vi "cs-scanning_v4_ssx.vi"() -> ()   [LabVIEW 2017]
uses:
  controls/boolean_info.ctl
  controls/z-axis-params_v4_prescan.ctl
  controls/TF-params.ctl
  fpga_subVIs_ssxy/fixed-point-ss/typeDefs/FXPControlParams_distEst.ctl
  <vilib>/Platform/TimedLoop/XDataNode/timing_clust.ctl
  <vilib>/Platform/TimedLoop/XDataNode/nitl_modes.ctl
  <vilib>/Platform/TimedLoop/XDataNode/wakeup.ctl
  <vilib>/rvi/Emulation/niFpgaSctlEmulationGetInTimedLoop.vi
  <vilib>/rvi/Emulation/niFpgaProcessEmulError.vi
  <vilib>/rvi/Emulation/niFpgaEmulationReportErrorSimple.vi
  <vilib>/rvi/Emulation/niFpgaGetClockAttributes.vi
  <vilib>/rvi/Emulation/niFpgaCriticalErrorInLSC.vi
  <vilib>/rvi/Memory/Memory_Emulation/nirvimemoryFastEmulation.vi
  <vilib>/rvi/Memory/Memory_Emulation/nirvimemoryEmulation.vi
  <vilib>/rvi/Emulation/niFpgaEmulationIsFPGAContextNoSignature.vi
  <vilib>/rvi/DataTransferAndStorage/Container/Common/niFpgaContainerGetUniqueNameForEmu.vi
  <vilib>/rvi/errors/nirviReportUnexpectedCaseInternalError (U32).vi
  <vilib>/rvi/eio/common/nirviEmuTemplateMethod_errors.vi
  <vilib>/rvi/Memory/Memory_Emulation/niFpgaMemoryEmulationCacheClearOnFirstRun.vi
  <vilib>/rvi/Memory/Memory_Emulation/nirvimemoryEmulationManagerCache_MakeExclusive.vi
  <vilib>/rvi/Memory/Memory_Emulation/niFpgaMemoryEmulationValidateCache.vi
  <vilib>/rvi/Memory/Memory_Emulation/nirvimemoryEmulationManagerCache_InsertValue.vi
  <vilib>/Utility/error.llb/Clear Errors.vi
  <vilib>/rvi/Memory/Memory_Emulation/nirvimemoryEmulationManagerCache_ReleaseExclusive.vi
  <vilib>/rvi/Memory/Memory_Emulation/nirvimemoryEmulationManagerCache_GetValue.vi
  <vilib>/rvi/Memory/Memory_Emulation/nirvimemoryEmulationManagerCache_SetValue.vi
  <vilib>/Platform/TimedLoop/XDataNode/XDataNode.xnode
  <vilib>/rvi/DataTransferAndStorage/Container/XNode/niFpgaContainer.xnode
  <vilib>/eio/EIONode/EIONode.xnode
  <vilib>/rvi/DataTransferAndStorage/Register/Emulation/niFpgaRegisterEmulation.vi
  FPGA-data-logging.lvlib
  libimaging-cs.lvlib
  <vilib>/Platform/TimedLoop/XDataNode/XDNodeRunTimeDep.lvlib
panel:
  in  "num-log-channels":i32
  out "SS FIFO TimeOut?":bool
  in  "ControlParamsLin":T1={"umax"=3.0, "Ns_obs/cntrl"=0, "ref_f_VEC"=[0.0, 0.0], "du_max"=0.0, "Nbar"=0.0, "Nhyst"=0, "Nsat"=0, "Ndrift+1"=0}
  in  "z_axis_params":T2={"TOL"=0.3, "z_u_max"=5.0, "setpoint-scan"=0.0, "Ki-scan"=0.001, "uz_safe"=0.0, "Kiz_down"=0.001, "prescan-samples"=0, "setpoint-up"=0.0, "TF-params"={"TF-order"=0, "Num"=[0.0, 0.0, 0.0, 0.0, 0.0, 0.0, 0.0, 0.0, 0.0], "Den"=[0.0, 0.0, 0.0, 0.0, 0.0, 0.0, 0.0, 0.0, 0.0]}, "do-Dz"=FALSE, "PID-while-xy-move"=FALSE} {"prescan-samples" format="%#_13g"; "uz_safe" format="%#_13g"; "TOL" format="%#_13g"}
  in  "zup-err-threshold":fxp<+,24,5>=0.10000038146972656 format="%#_21g"
  out "stop_loops":bool
  out "xy_k":fxp<+/-,16,5>[](array[numeric])
  out "xy_ref":fxp<+/-,16,5>[](array[numeric])
  out "u_x saturated":bool
  out "u_y saturated":bool
  out "state1-count":u64
  out "state5-count":u64
  out "state4-count":u64
  out "state3-count":u64
  out "state2-count":u64
  in  "collect all":bool
  out "entity-index":i16
  in  "TsTicks":u32=1600
  out "number-settled-samples-Z":i16
  out "Current Case":u8
  out "boolean \nindicators":T4
  out "z-u(k)":sgl
  in  "ABORT":bool
  out "read fifo timeout":bool
  in  "numEntities":i16
  in  "trigger-0":bool
  out "number-settled-samples-y":i16
  out "number-settled-samples-x":i16
  in  "xy-error-threshold":sgl format="%#_13g"
  in  "settled-samples\nthreshold":i16
  in  "Ki-xy":sgl=0.001 format="%#_13g"
  # "- If collect all = fasle ,\nwe only collect measurement data.\n- If collect all = true, we collect everything."
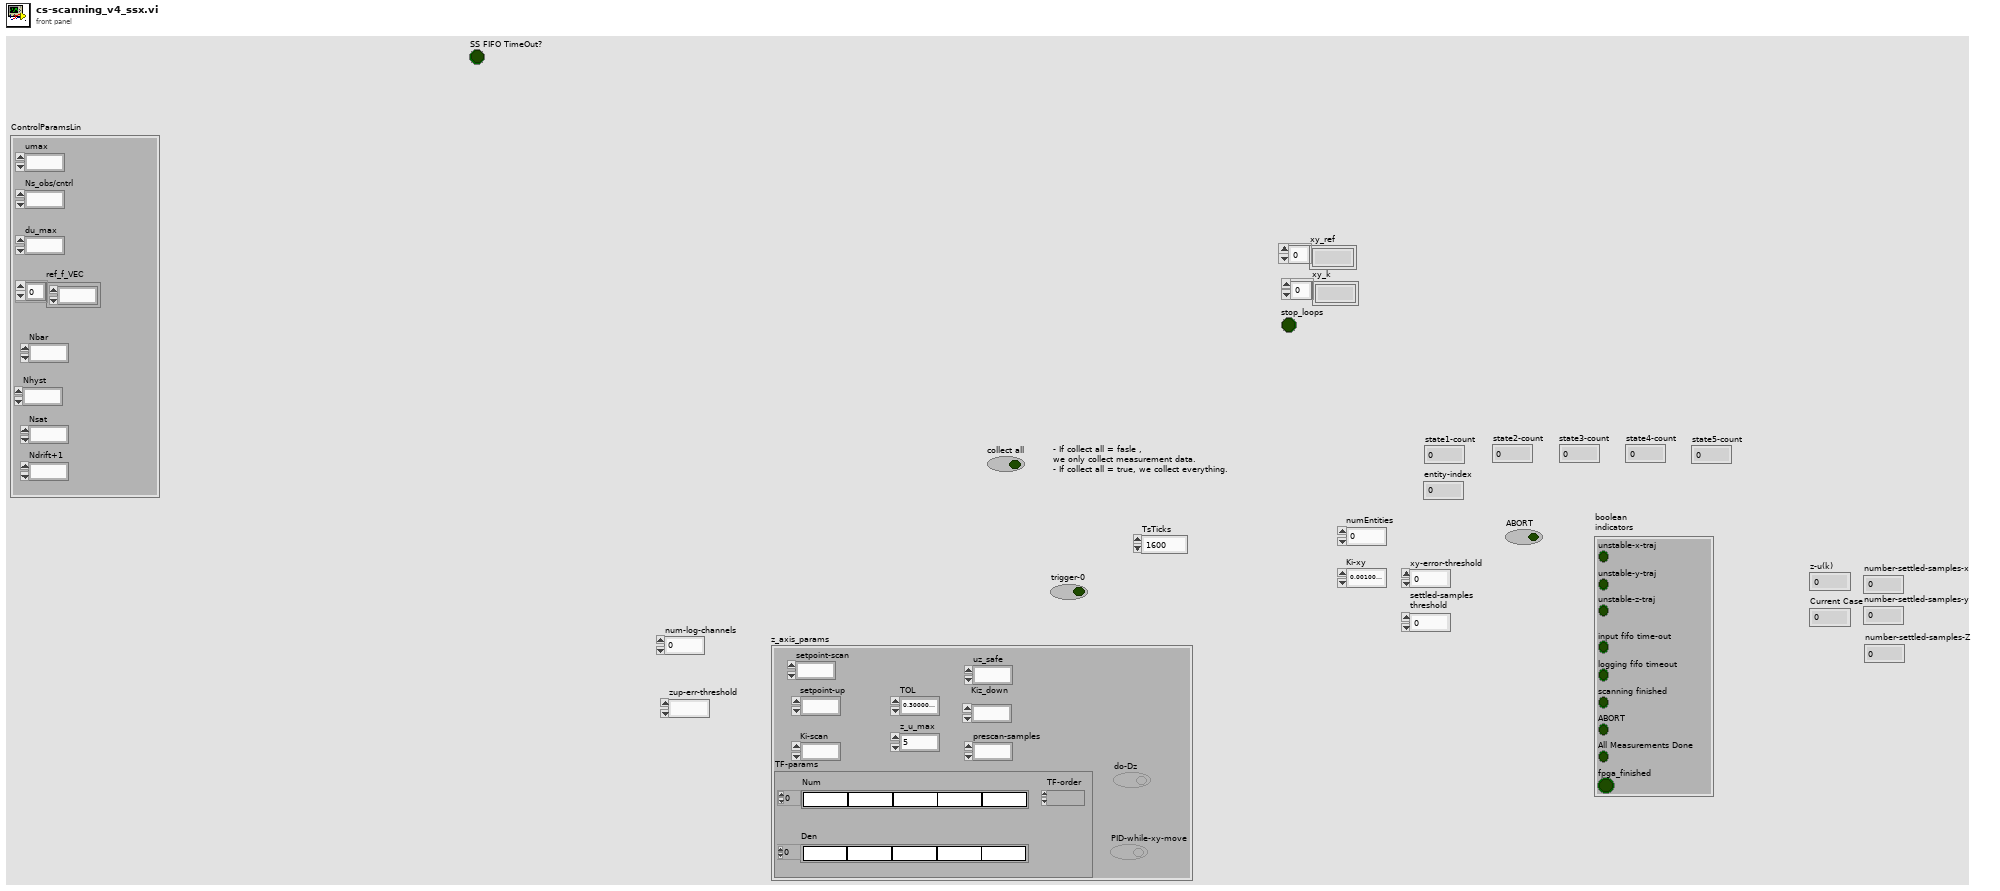
[diagram p1: front panel]
types:
  T1 = typedef "FXPControlParams_distEst.ctl" = cluster{"umax":fxp<+/-,18,5>, "Ns_obs/cntrl":u8, "ref_f_VEC":fxp<+/-,32,5>[], "du_max":fxp<+/-,18,5>, "Nbar":fxp<+/-,32,5>, "Nhyst":u8, "Nsat":u8, "Ndrift+1":u8}
  T2 = typedef "z-axis-params_v4_prescan.ctl" = cluster{"TOL":sgl, "z_u_max":sgl, "setpoint-scan":fxp<+/-,32,16>, "Ki-scan":sgl, "uz_safe":fxp<+/-,16,5>, "Kiz_down":sgl, "prescan-samples":i16, "setpoint-up":fxp<+/-,32,16>, "TF-params":T3, "do-Dz":bool, "PID-while-xy-move":bool}
  T3 = typedef "TF-params.ctl" = cluster{"TF-order":i16, "Num":sgl[], "Den":sgl[]}
  T4 = typedef "boolean_info.ctl" = cluster{"unstable-z-traj":bool, "input fifo time-out":bool, "logging fifo timeout":bool, "scanning finished":bool, "unstable-x-traj":bool, "unstable-y-traj":bool, "ABORT":bool, "All Measurements Done":bool, "fpga_finished":bool}
  T5 = typedef "XDNodeRunTimeDep.lvlib/timing_clust.ctl" = cluster{"Expected End [f-1]":u64, "Actual End [f-1]":u64, "Finished Late? [f-1]":bool, "Expected End [i-1]":u64, "Actual End [i-1]":u64, "Finished Late? [i-1]":bool, "Expected Start [i]":u64, "Actual Start [i]":u64, "Expected Start [f]":u64, "Actual Start [f]":u64, "Source Name":string, "Structure Name":string, "Period":i64, "Deadline":i64, "Offset":i64, "Start":i64, "Priority":i32, "Timeout":i32, "Mode":T6, "Wakeup Reason":T7, "Error":errorcluster, "Source Type":string, "Secondary Source Type":string, "Global End Time":u64, "Global Start Time":u64, "Frame Duration":u64, "Iteration Duration":u64, "Assigned CPU":i32, "I/O Scan Engine Mode":u32}
  T6 = typedef "XDNodeRunTimeDep.lvlib/nitl_modes.ctl" = enum32{"No Change", "Process missed periods, maintain original phase", "Discard missed periods, maintain original phase", "Process missed periods, ignore original phase", "Discard missed periods, ignore original phase"}
  T7 = typedef "XDNodeRunTimeDep.lvlib/wakeup.ctl" = enum32{"Normal", "Aborted", "Asynchronous wakeup", "Timing source error", "Timed loop error", "Timeout"}
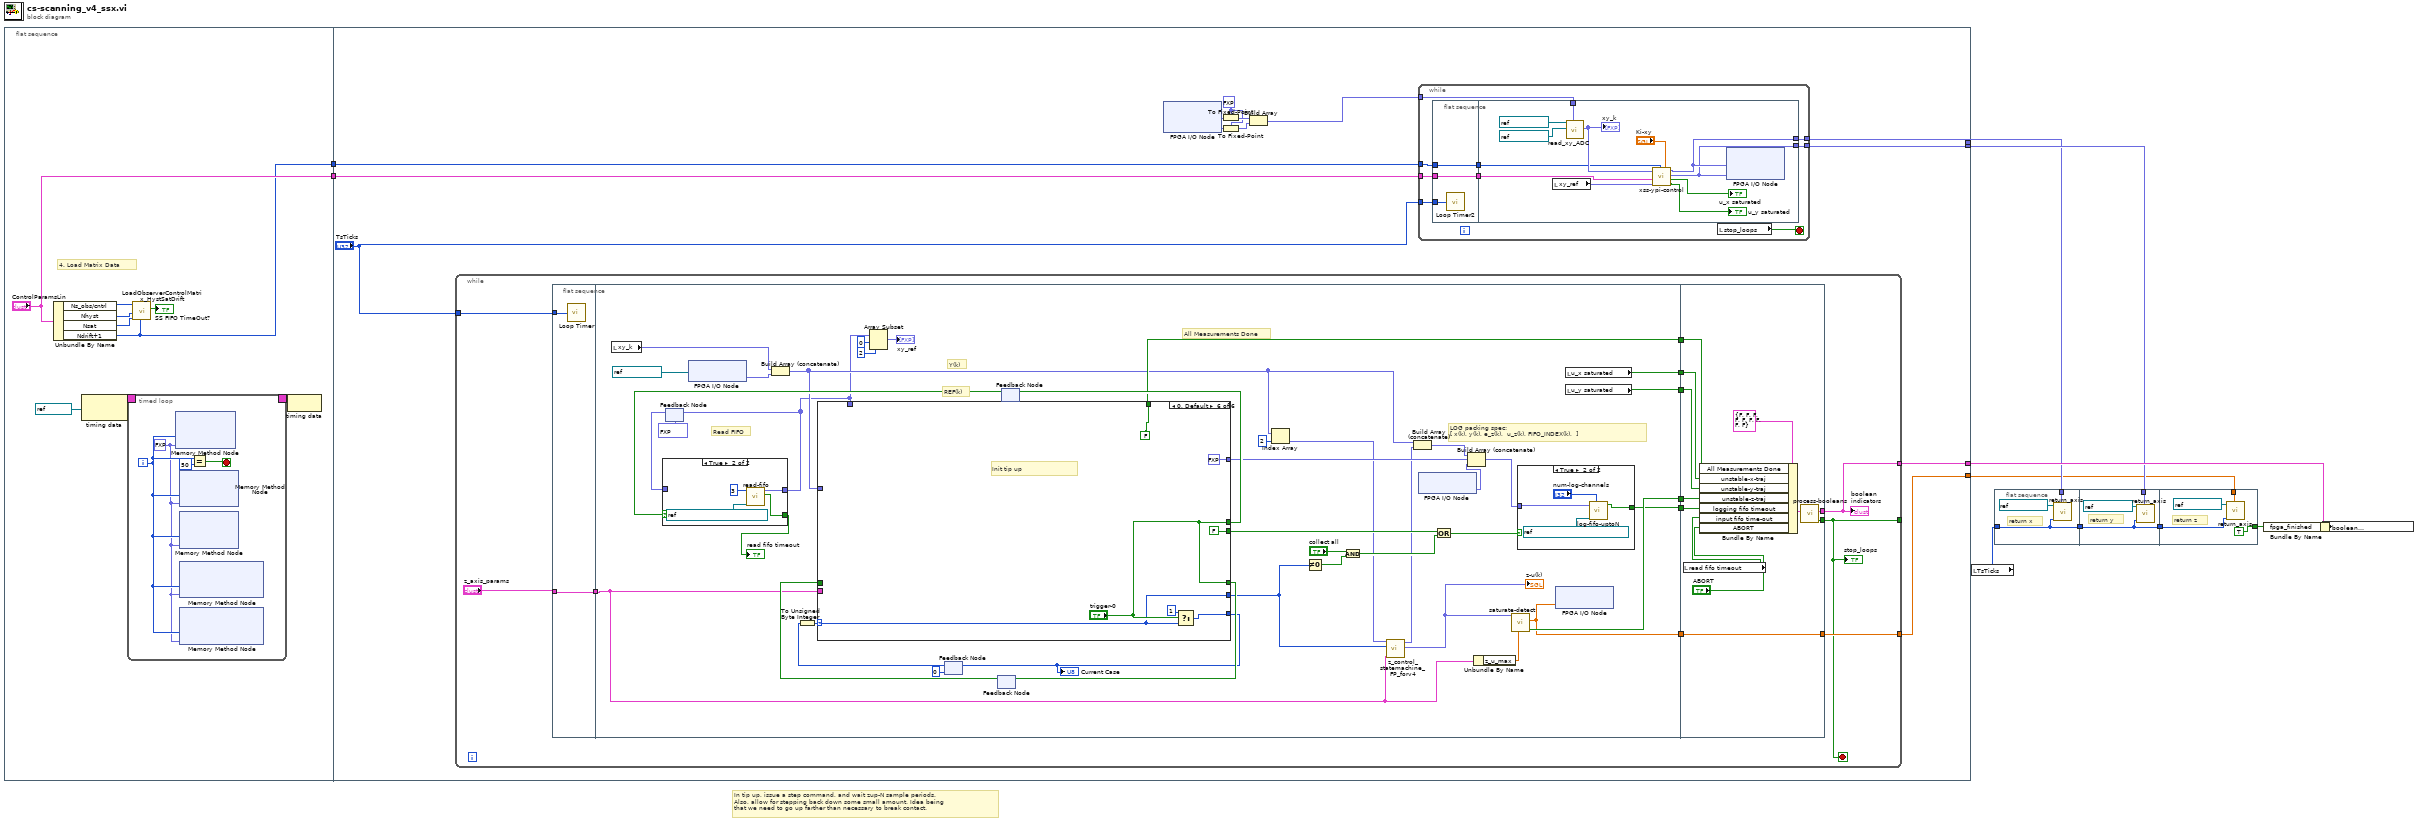
[diagram p0: block diagram]
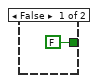
[diagram p2: hidden frame]
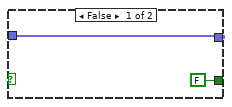
[diagram p3: hidden frame]
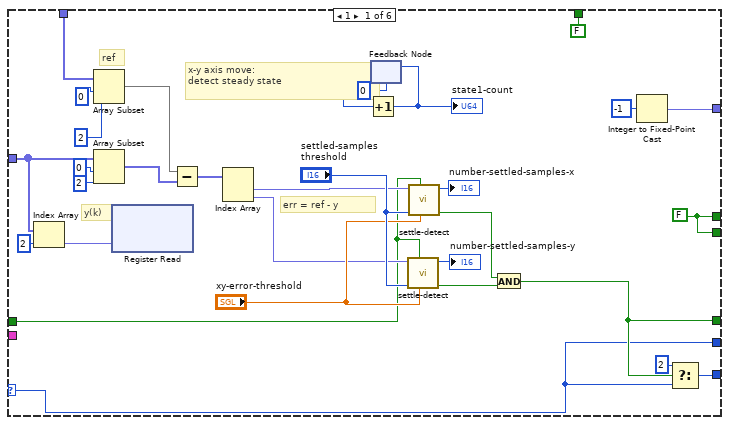
[diagram p4: hidden frame]
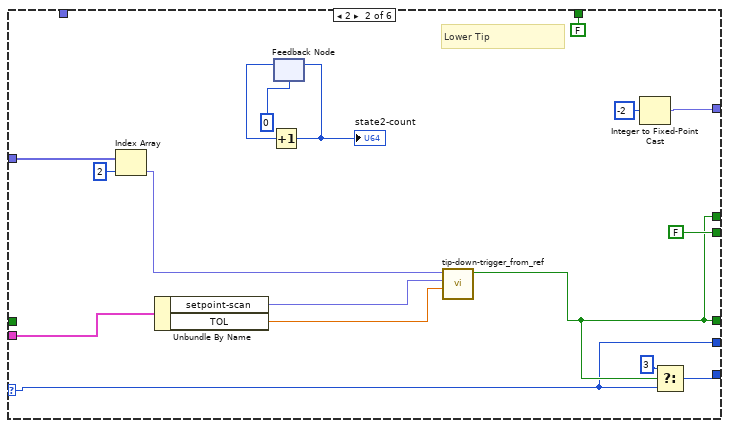
[diagram p5: hidden frame]
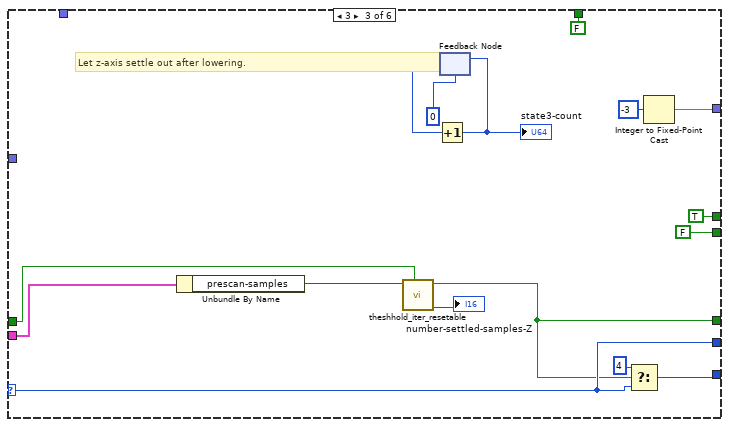
[diagram p6: hidden frame]
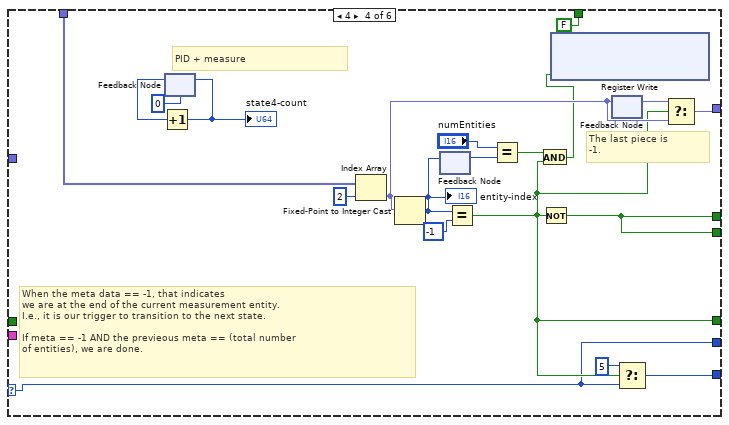
[diagram p7: hidden frame]
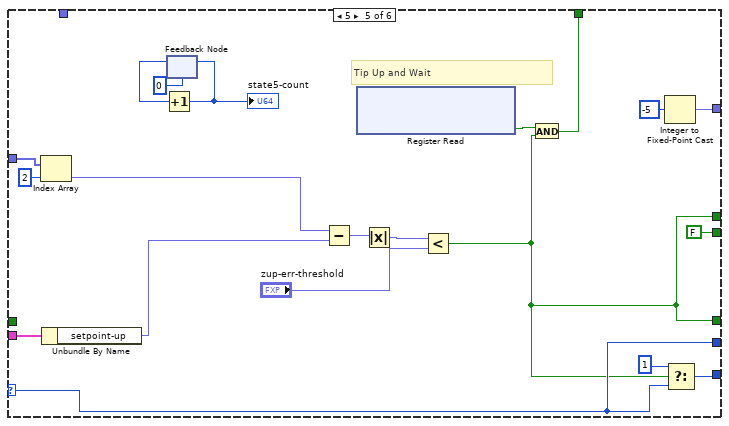
[diagram p8: hidden frame]
diagram:
  # "In tip up, issue a step command, and wait zup-N sample periods.\nAlso, allow for stepping back down some small amount. Idea being \nthat we need to go up farther than necessary to break contact."
  n1 = flat-sequence {
    tunnel: ["ControlParamsLin"] -> w2
    tunnel: [w12] -> w1
    tunnel: [w43] -> w9
    tunnel: [w41] -> w6
    tunnel: [w40] -> w5
    tunnel: [w39] -> w4
    tunnel: w2 -> [w32]
    tunnel: w1 -> [w31]
    frame #0 {
      # "4. Load Matrix Data"
      n2 = Unbundle By Name("ControlParamsLin") -> ("Ns_obs/cntrl"=w17:u8, "Nhyst"=w14:u8, "Nsat"=w13:u8, "Ndrift+1"=w12:u8)
      n3 = node-c288(refnum<k21> "80MHz" ("Source Name")) -> (w20:T5)
      n4 = timed-loop {
        timing: w20 -> [_]
        timing-out: [_] -> w19
        i -> [w22]
        stop <- w24 stop-if-true
        w21 = fxp<+/-,32,5> 0.0 ("Data")
        n5 = xnode ("Memory Method Node")("Address"=w22, "Data"=w21) -> ()  [unwired: 1 in, 1 out]
        n6 = xnode ("Memory Method Node")("Address"=w22, "Data"=w21) -> ()  [unwired: 1 in, 1 out]
        n7 = xnode ("Memory Method Node")("Address"=w22, "Data"=w21) -> ()  [unwired: 1 in, 1 out]
        n8 = xnode ("Memory Method Node")("Address"=w22, "Data"=w21) -> ()  [unwired: 1 in, 1 out]
        n9 = xnode ("Memory Method Node")("Address"=w22, "Data"=w21) -> ()  [unwired: 1 in, 1 out]
        n10 = Equal?(x=w22, y=50) -> (x = y?=w24:bool)
      }
      n11 = call "LoadObserverControlMatrix_HystSatDrift.vi"("Ndrift+1"=w12, "Nsat"=w13, "Nhyst"=w14, "NS_obs/cntrl"=w17) -> ("SS FIFO TimeOut?"=→"SS FIFO TimeOut?":bool)  [unwired: 7 in]
      n12 = node-c288(w19) -> ()
    }
    frame #1 {
      w34 = fxp<+/-,16,5> 0.0 ("fixed-point type")
      n13 = while {
        tunnel: "TsTicks" -> [w51]
        tunnel: [w47] -> _
        tunnel: [w49] -> w39
        tunnel: [w48] -> w43
        stop <- w47 stop-if-true
        n14 = flat-sequence {
          tunnel: w51 -> [w56]
          tunnel: "z_axis_params" -> [w57]
          tunnel: [w57] -> w55
          tunnel: w55 -> [w59]
          tunnel: [w96] -> w54
          tunnel: [w95] -> w53
          tunnel: [w83] -> w52
          tunnel: [w64] -> w50
          tunnel: [w78] -> w46
          tunnel: [w77] -> w45
          tunnel: w54 -> [w232]
          tunnel: w53 -> [w229]
          tunnel: w52 -> [w226]
          tunnel: [w225] -> w47
          tunnel: [w224] -> w48
          tunnel: [w223] -> w49
          tunnel: w50 -> [w223]
          tunnel: w46 -> [w222]
          tunnel: w45 -> [w221]
          frame #0 {
            n15 = call "Loop Timer"("Count(Ticks)"=w56) -> ()  [unwired: 1 out]
          }
          frame #1 {
            # "All Measurements Done"
            # "REF(k)"
            # "Y(k)"
            # "LOG packing spec:\n[ x(k), y(k), e_z(k),  u_z(k), FIFO_INDEX(k),  ]"
            # "Read FIFO"
            n16 = local read "xy_k"() -> (w70:fxp<+/-,16,5>[])
            n17 = feedback #1(fxp<+/-,16,5>[] [0.0, 0.0, 0.0] ("unpacked-data")) -> (w98:fxp<+/-,16,5>[])
            n18 = xnode "FPGA I/O Node"("FPGA I/O In"=refnum<k21> "Mod2/AI2" ("y - ADC")) -> ("I/O Item"=w74:fxp<+/-,24,5>)  [unwired: 1 out]
            n19 = Build Array (concatenate)(w70, w74) -> (w73:fxp<+/-,24,5>[])
            n20 = feedback #2(u8 0 ("t")) -> (w68:u8)
            n21 = To Unsigned Byte Integer(number=w68) -> (unsigned 8bit integer=w69:u8)
            n22 = feedback #3() -> (w89:bool)  [unwired: 1 in]
            n23 = feedback #4() -> (w92:bool)  [unwired: 1 in]
            n24 = case shown="True" w92 {
              tunnel: w98 -> [w105 _]
              tunnel: [w105 w107] -> w65
              tunnel: [FALSE ("timout?") w106] -> w94
              frame False {
              }
              frame True {
                n25 = call "read-fifo.vi"("FIFO In"=refnum<k21> "host-to-fpga-fxp-16-5", "numChan"=3) -> ("timout?"=w106:bool, "unpacked-data"=w107:fxp<+/-,16,5>[])  [unwired: 8 in]
              }
            }
            "read fifo timeout" <- w94
            n26 = feedback-in #1(w65) -> ()
            n27 = case shown="0, Default" w69 {
              selector: w69 -> [w110 w141 w162 w174 w201 w214]
              tunnel: [w111 FALSE FALSE ("trigger-0") w184 FALSE FALSE] -> w84
              tunnel: [w133 w153 w172 w192 w212 w220] -> w67
              tunnel: w73 -> [w112 w155 _ _ w203 _]
              tunnel: [w111 w143 TRUE ("trigger-0") w184 w196 "trigger-0"] -> w93
              tunnel: w59 -> [_ w157 w170 _ w195 _]
              tunnel: [FALSE FALSE FALSE FALSE w205 FALSE] -> w83
              tunnel: w65 -> [w124 _ _ w186 _ _]
              tunnel: w89 -> [w122 _ w163 _ _ _]
              tunnel: [w121 w143 w159 w177 w196 "trigger-0"] -> w90
              tunnel: [w115 w144 w164 w180 w206 fxp<+/-,16,5> 0.0 ("Element")] -> w71
              tunnel: [w110 w141 w162 w174 w201 w214] -> w62
              frame 1 {
                w111 = FALSE
                # "y(k)"
                # "err = ref - y"
                # "ref"
                # "x-y axis move: \ndetect steady state"
                n28 = Index Array(array=w112, index=2) -> (element=w114:fxp<+/-,24,5>)
                n29 = Array Subset(array=w124, index=0, length=2) -> (w128:fxp<+/-,16,5>[])
                n30 = Array Subset(array=w112, index=0, length=2) -> (w127:fxp<+/-,24,5>[])
                n31 = xnode ("Register Read")("Data"=w114) -> ()  [unwired: 1 in, 1 out]
                n32 = Subtract(x=w128, y=w127) -> (x-y=w120:fxp<+/-,25,6>[])
                n33 = Index Array(array=w120) -> (element #1=w126:fxp<+/-,25,6>, element #2=w125:fxp<+/-,25,6>)  [unwired: 2 in]
                n34 = feedback #5(u64 0) -> (w118:u64)
                n35 = Increment(x=w118) -> (x+1=w119:u64)
                "state1-count" <- w119
                n36 = feedback-in #5(w119) -> ()
                n37 = call "settle-detect.vi"("error-max"="xy-error-threshold", "reset"=w122, "settled-samples\nthreshold"="settled-samples\nthreshold", "err(k)"=w125) -> ("has-settled"=w140:bool, "number-settled-samples"=→"number-settled-samples-y":u16)  [unwired: 6 in]
                n38 = call "settle-detect.vi"("error-max"="xy-error-threshold", "reset"=w122, "settled-samples\nthreshold"="settled-samples\nthreshold", "err(k)"=w126) -> ("has-settled"=w139:bool, "number-settled-samples"=→"number-settled-samples-x":u16)  [unwired: 6 in]
                n39 = And(x=w139, y=w140) -> (x .and. y?=w121:bool)
                n40 = Integer to Fixed-Point Cast(integer=i16 -1) -> (fixed-point=w115:fxp<+/-,16,5>)  [unwired: 1 in]
                n41 = Select(t=u8 2, s=w121, f=w110) -> (s? t:f=w133:u8)
              }
              frame 2 {
                # "Lower Tip"
                n42 = Index Array(array=w155, index=2) -> (element=w154:fxp<+/-,24,5>)
                n43 = Unbundle By Name(w157) -> ("setpoint-scan"=w145:fxp<+/-,32,16>, "TOL"=w142:sgl)
                n44 = feedback #6(u64 0) -> (w148:u64)
                n45 = Increment(x=w148) -> (x+1=w149:u64)
                "state2-count" <- w149
                n46 = feedback-in #6(w149) -> ()
                n47 = call "tip-down-trigger_from_ref.vi"("TOL"=w142, "setpoint"=w145, "I/O Item"=w154) -> ("Boolean"=w143:bool)  [unwired: 8 in]
                n48 = Integer to Fixed-Point Cast(integer=i16 -2) -> (fixed-point=w144:fxp<+/-,16,5>)  [unwired: 1 in]
                n49 = Select(t=u8 3, s=w143, f=w141) -> (s? t:f=w153:u8)
              }
              frame 3 {
                # "Let z-axis settle out after lowering."
                n50 = Unbundle By Name(w170) -> ("prescan-samples"=w161:i16)
                n51 = call "theshhold_iter_resetable.vi"("reset"=w163, "N"=w161) -> ("iter"=→"number-settled-samples-Z":i16, "Boolean"=w159:bool)  [unwired: 8 in]
                n52 = feedback #7(u64 0) -> (w167:u64)
                n53 = Increment(x=w167) -> (x+1=w168:u64)
                "state3-count" <- w168
                n54 = feedback-in #7(w168) -> ()
                n55 = Select(t=u8 4, s=w159, f=w162) -> (s? t:f=w172:u8)
                n56 = Integer to Fixed-Point Cast(integer=i16 -3) -> (fixed-point=w164:fxp<+/-,16,5>)  [unwired: 1 in]
              }
              frame 4 {
                # "The last piece is\n-1."
                # "When the meta data == -1, that indicates\nwe are at the end of the current measurement entity.\nI.e., it is our trigger to transition to the next state.\n\nIf meta == -1 AND the previeous meta == (total number\nof entities), we are done."
                # "PID + measure"
                n57 = feedback #8(u64 0) -> (w182:u64)
                n58 = Increment(x=w182) -> (x+1=w183:u64)
                "state4-count" <- w183
                n59 = feedback-in #8(w183) -> ()
                n60 = Index Array(array=w186, index=2) -> (element=w178:fxp<+/-,16,5>)
                n61 = Fixed-Point to Integer Cast(1:w178) -> (0:w185:i16)
                "entity-index" <- w185
                n62 = feedback #9() -> (w187:i16)  [unwired: 1 in]
                n63 = feedback-in #9(w185) -> ()
                n64 = Equal?(x=w185, y=i16 -1) -> (x = y?=w177:bool)
                n65 = Equal?(x="numEntities", y=w187) -> (x = y?=w188:bool)
                n66 = And(x=w188, y=w177) -> (x .and. y?=w176:bool)
                n67 = Not(x=w177) -> (.not. x?=w184:bool)
                n68 = xnode ("Register Write")("Data"=w176) -> ()  [unwired: 1 in, 1 out]
                n69 = feedback #10() -> (w179:fxp<+/-,16,5>)  [unwired: 1 in]
                n70 = feedback-in #10(w178) -> ()
                n71 = Select(t=u8 5, s=w177, f=w174) -> (s? t:f=w192:u8)
                n72 = Select(t=w179, s=w177, f=w178) -> (s? t:f=w180:fxp<+/-,16,5>)
              }
              frame 5 {
                # "Tip Up and Wait"
                n73 = Index Array(array=w203, index=2) -> (element=w200:fxp<+/-,24,5>)
                n74 = Unbundle By Name(w195) -> ("setpoint-up"=w194:fxp<+/-,32,16>)
                n75 = feedback #11(u64 0) -> (w209:u64)
                n76 = Increment(x=w209) -> (x+1=w210:u64)
                "state5-count" <- w210
                n77 = feedback-in #11(w210) -> ()
                n78 = Subtract(x=w200, y=w194) -> (x-y=w199:fxp<+/-,36,17>)
                n79 = xnode ("Register Read")() -> ("Data"=w202:bool)  [unwired: 1 in, 1 out]
                n80 = Absolute Value(x=w199) -> (abs(x)=w198:fxp<+,35,16>)
                n81 = Less?(x=w198, y="zup-err-threshold") -> (x < y?=w196:bool)
                n82 = And(x=w202, y=w196) -> (x .and. y?=w205:bool)
                n83 = Integer to Fixed-Point Cast(integer=i16 -5) -> (fixed-point=w206:fxp<+/-,16,5>)  [unwired: 1 in]
                n84 = Select(t=u8 1, s=w196, f=w201) -> (s? t:f=w212:u8)
              }
              frame 0, Default {
                # "Init tip up"
                n85 = Select(t=u8 1, s="trigger-0", f=w214) -> (s? t:f=w220:u8)
              }
            }
            "Current Case" <- w67
            n86 = Array Subset(array=w65, index=0, length=2) -> (→"xy_ref":fxp<+/-,16,5>[])
            n87 = feedback-in #2(w67) -> ()
            n88 = feedback-in #3(w90) -> ()
            n89 = feedback-in #4(w93) -> ()
            n90 = Index Array(array=w73, index=2) -> (element=w61:fxp<+/-,24,5>)
            n91 = Not Equal To 0?(x=w62) -> (x != 0?=w87:bool)
            n92 = And(x="collect all", y=w87) -> (x .and. y?=w85:bool)
            n93 = call "z_control_statemachine_FP_forv4.vi"("z_axis_params"=w59, "State"=w62, "zerr(k)"=w61) -> ("zuk_Dinv"=w63:fxp<+/-,16,5>, "z-u(k)"=w60:fxp<+/-,16,5>)  [unwired: 7 in]
            "z-u(k)" <- w63
            n94 = Build Array (concatenate)(w73, w60) -> (w72:fxp<+/-,24,5>[])
            n95 = xnode "FPGA I/O Node"() -> ("Mod2/AI3"=w58:fxp<+/-,24,5>)  [unwired: 1 in, 1 out]
            n96 = Or(x=w84, y=w85) -> (x .or. y?=w88:bool)
            n97 = Build Array (concatenate)(w72, w71, w58) -> (w97:fxp<+/-,24,5>[])
            n98 = Unbundle By Name(w59) -> ("z_u_max"=w81:sgl)
            n99 = call "saturate-detect.vi"("bound"=w81, "x"=w63) -> ("saturated"=w96:bool, "sat(x)"=w64:sgl)  [unwired: 8 in]
            n100 = case shown="True" w88 {
              tunnel: w97 -> [_ w103]
              tunnel: [FALSE ("logging-timeout?") w102] -> w95
              frame False {
              }
              frame True {
                n101 = call "log-fifo-uptoN.vi"("N"="num-log-channels", "FIFO In"=refnum<k21> "fpga-to-host2-fxp-16-5", "input-data"=w103) -> ("logging-timeout?"=w102:bool)  [unwired: 8 in]
              }
            }
            n102 = xnode "FPGA I/O Node"("Mod1/AO2"=w64) -> ()  [unwired: 1 in, 1 out]
            n103 = local read "u_x saturated"() -> (w78:bool)
            n104 = local read "u_y saturated"() -> (w77:bool)
          }
          frame #2 {
            n105 = local read "read fifo timeout"() -> (w228:bool)
            n106 = Bundle By Name(cluster=T4 {"unstable-z-traj"=FALSE, "input fifo time-out"=FALSE, "logging fifo timeout"=FALSE, "scanning finished"=FALSE, "unstable-x-traj"=FALSE, "unstable-y-traj"=FALSE, "ABORT"=FALSE, "All Measurements Done"=FALSE, "fpga_finished"=FALSE} ("boolean errors"), "All Measurements Done"=w226, "unstable-x-traj"=w222, "unstable-y-traj"=w221, "unstable-z-traj"=w232, "logging fifo timeout"=w229, "input fifo time-out"=w228, "ABORT"="ABORT") -> (w230:T4)
            n107 = call "process-booleans.vi"("boolean indicators 2"=w230) -> ("scaning finished"=w225:bool, "boolean indicators"=w224:T4)  [unwired: 9 in]
          }
        }
        "boolean \nindicators" <- w48
        "stop_loops" <- w47
      }
      n108 = xnode "FPGA I/O Node"() -> ("Mod2/AI0"=w37:fxp<+/-,24,5>, "Mod2/AI1"=w35:fxp<+/-,24,5>)  [unwired: 2 in, 2 out]
      n109 = To Fixed-Point(fixed-point type=w34, number=w37) -> (fixed-point=w38:fxp<+/-,16,5>)
      n110 = To Fixed-Point(fixed-point type=w34, number=w35) -> (fixed-point=w36:fxp<+/-,16,5>)
      n111 = Build Array(w38, w36) -> (w33:fxp<+/-,16,5>[])
      n112 = while {
        tunnel: "TsTicks" -> [w241]
        tunnel: [w240] -> w41
        tunnel: [w239] -> w40
        tunnel: w33 -> [w237]
        tunnel: w32 -> [w235]
        tunnel: w31 -> [w233]
        stop <- w238 stop-if-true
        n113 = flat-sequence {
          tunnel: w241 -> [w244]
          tunnel: [w243] -> w236
          tunnel: w235 -> [w243]
          tunnel: w233 -> [w242]
          tunnel: [w242] -> w234
          tunnel: [w248] -> w240
          tunnel: [w249] -> w239
          tunnel: w237 -> [w254]
          tunnel: w236 -> [w250]
          tunnel: w234 -> [w245]
          frame #0 {
            n114 = call "Loop Timer2"("Count(Ticks)"=w244) -> ()  [unwired: 1 out]
          }
          frame #1 {
            n115 = local read "xy_ref"() -> (w253:fxp<+/-,16,5>[])
            n116 = call "read_xy_ADC.vi"("x(0), y(0)"=w254, "y - ADC"=refnum<k21> "Mod2/AI1", "x - ADC"=refnum<k21> "Mod2/AI0") -> ("x_y"=w252:fxp<+/-,17,6>[])  [unwired: 8 in]
            "xy_k" <- w252
            n117 = call "xss-ypi-control.vi"("Ki-xy"="Ki-xy", "Ns_nsw"=w245, "xy-ref"=w253, "ControlParamsLin"=w250, "x_k-y_k"=w252) -> ("u_y saturated"=→"u_y saturated":bool, "u_x saturated"=→"u_x saturated":bool, "sat(u_y)"=w248:fxp<+/-,18,5>, "u_k (saturated)"=w249:fxp<+/-,32,5>)  [unwired: 3 in]
            n118 = xnode "FPGA I/O Node"("Mod1/AO0"=w249, "Mod1/AO1"=w248) -> ()  [unwired: 2 in, 2 out]
          }
        }
        n119 = local read "stop_loops"() -> (w238:bool)
      }
    }
  }
  n120 = local read "TsTicks"() -> (w3:u32)
  n121 = flat-sequence {
    tunnel: w3 -> [w258]
    tunnel: w5 -> [w259]
    tunnel: [w258] -> w11
    tunnel: w6 -> [w262]
    tunnel: w11 -> [w260]
    tunnel: [w260] -> w10
    tunnel: w4 -> [w266]
    tunnel: w10 -> [w264]
    tunnel: [TRUE] -> w8
    frame #0 {
      # "return x"
      n122 = call "return_axis.vi"("u(0)"=w259, "TsTicks"=w258, "FPGA I/O In"=refnum<k21> "Mod1/AO0") -> ()  [unwired: 9 in]
    }
    frame #1 {
      # "return y"
      n123 = call "return_axis.vi"("u(0)"=w262, "TsTicks"=w260, "FPGA I/O In"=refnum<k21> "Mod1/AO1") -> ()  [unwired: 9 in]
    }
    frame #2 {
      # "return z"
      n124 = call "return_axis.vi"("u(0)"=w266, "TsTicks"=w264, "FPGA I/O In"=refnum<k21> "Mod1/AO2") -> ()  [unwired: 9 in]
    }
  }
  n125 = Bundle By Name(cluster=w9, "fpga_finished"=w8) -> (w7:T4)
  n126 = local write "boolean \nindicators"(w7) -> ()
